vi "DMA to Transfer.vi"(8 "error in (no error)":errorcluster, 9 "Transfer in":refnum<class "Transfer.lvclass">, 10 "DMA Transfer Spec in":T1 {"Block Descriptors"."descriptor params"."data ptr (lower)" format="%.0x"; "Block Descriptors"."descriptor params"."data ptr (upper)" format="%.0x"; "Block Descriptors"."descriptor params"."data size" format="%.0x"; "Block Descriptors"."descriptor params"."next descriptor ptr" format="%.0x"; "Block Descriptors"."descriptor size" format="%08x"; "Block Descriptors"."descriptor ptr (RFM)" format="%08x"; "Block Descriptors"."descriptor ptr (VISA)" format="%08x"; "RFM offset" format="%08x"}, 11 "GE 5565PIORC in":refnum<class "GE 5565PIORC.lvclass">) -> (0 "error out":errorcluster, 1 "Transfer out":refnum<class "Transfer.lvclass">, 2 "DMA Transfer Spec out":T1 {"Block Descriptors"."descriptor params"."data ptr (lower)" format="%.0x"; "Block Descriptors"."descriptor params"."data ptr (upper)" format="%.0x"; "Block Descriptors"."descriptor params"."data size" format="%.0x"; "Block Descriptors"."descriptor params"."next descriptor ptr" format="%.0x"; "Block Descriptors"."descriptor size" format="%08x"; "Block Descriptors"."descriptor ptr (RFM)" format="%08x"; "Block Descriptors"."descriptor ptr (VISA)" format="%08x"; "RFM offset" format="%08x"}, 3 "GE 5565PIORC out":refnum<class "GE 5565PIORC.lvclass">)   [LabVIEW 2017, in "GE Reflective Memory.lvlib" / "GE Reflective Memory Transceiver.lvclass"]
uses:
  GE Reflective Memory Transceiver.lvclass
  <vilib>/NI/GE Reflective Memory Driver/Typedefs/GE 5565PIORC.Typedef.DMA Transfer Spec.ctl
  <vilib>/NI/GE Reflective Memory Driver/Typedefs/GE 5565PIORC.Typedef.DMA Block Descriptor.ctl
  <vilib>/NI/GE Reflective Memory Driver/Typedefs/GE 5565PIORC.Typedef.DMA Block Descriptor Params.ctl
  Builds/Data Sharing Framework/Current/Core/DSF Core.lvlibp/Classes/Transfer/Transfer.lvclass
  <vilib>/NI/GE Reflective Memory Driver/GE 5565PIORC.lvclass
  <vilib>/NI/GE Reflective Memory Driver/GE 5565PIORC.lvclass/GE 5565PIORC.ctl
  <vilib>/NI/GE Reflective Memory Driver/Methods/GE 5565PIORC.DMA.Get Transfer Components (Block).vi
  <vilib>/NI/GE Reflective Memory Driver/Methods/GE 5565PIORC.DMA.Block.Read (Pointer).vi
  <vilib>/NI/GE Reflective Memory Driver/Methods/GE 5565PIORC.VISA.Move In.Pointer (MEMACC).vi
  <vilib>/NI/GE Reflective Memory Driver/Methods/GE 5565PIORC.VISA.Return Handler.vi
  <vilib>/Utility/error.llb/Error Cluster From Error Code.vi
  Builds/Data Sharing Framework/Current/Core/DSF Core.lvlibp/Classes/Buffer/Buffer.lvclass
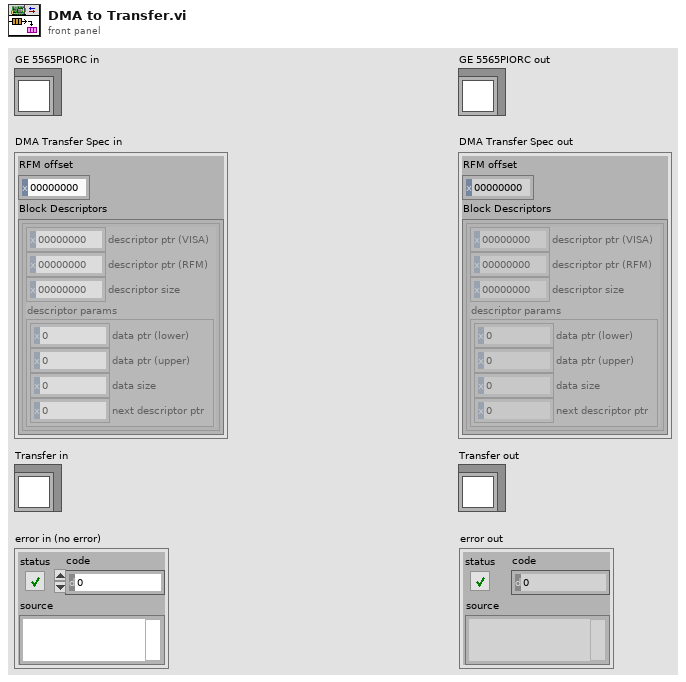
[diagram p1: front panel]
types:
  T1 = typedef "GE 5565PIORC.lvclass/GE 5565PIORC.Typedef.DMA Transfer Spec.ctl" = cluster{"RFM offset":u32, "Block Descriptors":T2[]}
  T2 = typedef "GE 5565PIORC.lvclass/GE 5565PIORC.Typedef.DMA Block Descriptor.ctl" = cluster{"descriptor ptr (VISA)":u32, "descriptor ptr (RFM)":u32, "descriptor size":u32, "descriptor params":T3}
  T3 = typedef "GE 5565PIORC.lvclass/GE 5565PIORC.Typedef.DMA Block Descriptor Params.ctl" = cluster{"data ptr (lower)":u32, "data ptr (upper)":u32, "data size":u32, "next descriptor ptr":u32}
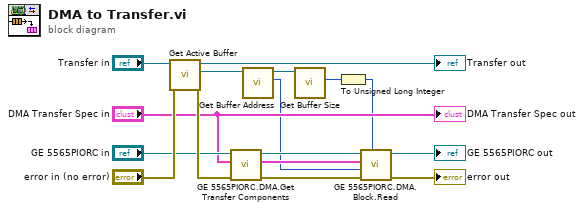
[diagram p0: block diagram]
diagram:
  n1 = call "Get Active Buffer.vi"("error in (no error)"="error in (no error)", "Transfer in"="Transfer in") -> ("error out"=w16:errorcluster, "Buffer"=w1:refnum<class "Buffer.lvclass">, "Transfer out"=→"Transfer out":refnum<class "Transfer.lvclass">)  [unwired: 7 in]
  n2 = call-poly <vilib>:"GE 5565PIORC.DMA.Get Transfer Components.vi"("error in (no error)"=w16, "DMA Transfer Spec in"="DMA Transfer Spec in", "GE 5565PIORC in"="GE 5565PIORC in") -> ("error out"=w11:errorcluster, "Block Descriptor"=w14:T2, "GE 5565PIORC out"=w13:refnum<class "GE 5565PIORC.lvclass">)  [unwired: 5 in, 1 out]
  n3 = call "Get Buffer Address.vi"("Buffer in"=w1) -> ("buffer address"=w4:u64, "Buffer out"=w5:refnum<class "Buffer.lvclass">)  [unwired: 9 in]
  n4 = call "Get Buffer Size.vi"("Buffer in"=w5) -> ("buffer size"=w12:u64)  [unwired: 9 in, 1 out]
  n5 = To Unsigned Long Integer(number=w12) -> (unsigned 32bit integer=w6:u32)
  n6 = call-poly <vilib>:"GE 5565PIORC.DMA.Block.Read.vi"("bytes to move"=w6, "error in (no error)"=w11, "dst pointer"=w4, "Block Descriptor in"=w14, "GE 5565PIORC in"=w13) -> ("error out"=→"error out":errorcluster, "GE 5565PIORC out"=→"GE 5565PIORC out":refnum<class "GE 5565PIORC.lvclass">)  [unwired: 3 in, 2 out]
  "DMA Transfer Spec out" <- "DMA Transfer Spec in"
